vi "creat part type file.vi"() -> (3 "new file path (Not A Path if cancelled)":path caption="新建文件路径（取消时为非法路径）")   [LabVIEW 2018]
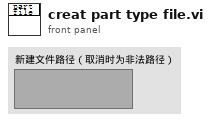
[diagram p1: front panel]
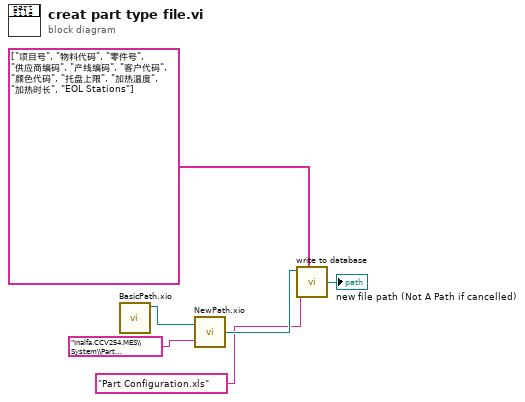
[diagram p0: block diagram]
diagram:
  n1 = call "BasicPath.xio.vi"() -> ("stripped path"=w6:path)  [unwired: 10 in, 1 out]
  n2 = call "NewPath.xio.vi"("Append path"="Inalfa.CCV254.MES\\System\\Part Configuration", "Basic path"=w6) -> ("New path"=w4:path)
  n3 = call "write to database.vi"("Header"=string[] ["项目号", "物料代码", "零件号", "供应商编码", "产线编码", "客户代码", "颜色代码", "托盘上限", "加热温度", "加热时长", "EOL Stations"], "file name"="Part Configuration.xls", "path"=w4) -> ("new file path (Not A Path if cancelled)"=→"new file path (Not A Path if cancelled)":path)  [unwired: 3 in]
